vi "rand generator.vi"() -> ()   [LabVIEW 2012]
panel:
  out "s? t:f":dbl
  out "number (0 to 1)":dbl
  in  "millisecond multiple":u32=1000
  out "Boolean":bool
  in  "stop":bool
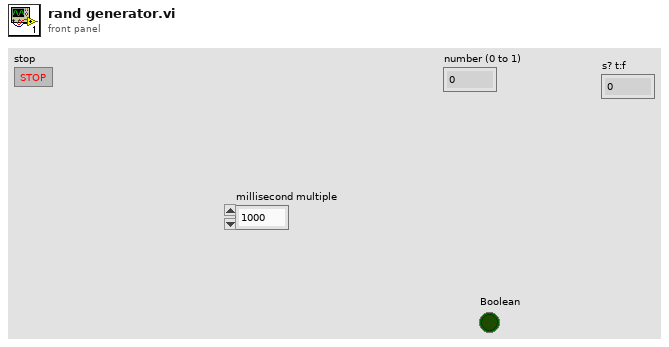
[diagram p1: front panel]
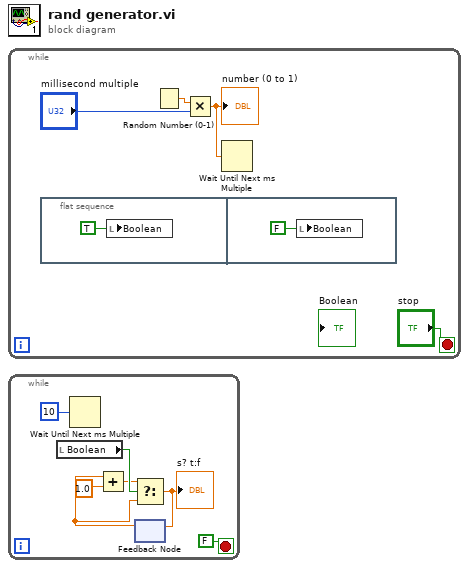
[diagram p0: block diagram]
diagram:
  n1 = while {
    stop <- "stop" stop-if-true
    n2 = flat-sequence {
      frame #0 {
        n3 = local write "Boolean"(TRUE) -> ()
      }
      frame #1 {
        n4 = local write "Boolean"(FALSE) -> ()
      }
    }
    n5 = Random Number (0-1)() -> (number: 0 to 1=w2:dbl)
    n6 = Multiply(x=w2, y="millisecond multiple") -> (x*y=w1:dbl)
    "number (0 to 1)" <- w1
    n7 = Wait Until Next ms Multiple(millisecond multiple=w1) -> ()  [unwired: 1 out]
  }
  n8 = while {
    stop <- FALSE stop-if-true
    n9 = local read "Boolean"() -> (w12:bool)
    n10 = Wait Until Next ms Multiple(millisecond multiple=u32 10) -> ()  [unwired: 1 out]
    n11 = feedback #1() -> (w8:dbl)  [unwired: 1 in]
    n12 = Add(x=w8, y=1.0) -> (x+y=w9:dbl)
    n13 = Select(t=w9, s=w12, f=w8) -> (s? t:f=w11:dbl)
    "s? t:f" <- w11
    n14 = feedback-in #1(w11) -> ()
  }
